vi "Init.vi"(8 "error in (no error)":errorcluster, 10 "Size":cluster{"Width":u16, "Height":u16}, 11 "Class 1 in":refnum<class "Freetype Drawer.lvclass">) -> (0 "error out":errorcluster, 3 "Class 1 out":refnum<class "Freetype Drawer.lvclass">)   [LabVIEW 2023, in "Freetype Drawer.lvlib" / "Freetype Drawer.lvclass"]
uses:
  Freetype Drawer.lvclass
  Freetype Drawer.lvclass/Freetype Drawer.ctl
  Freetype Drawer.lvlib
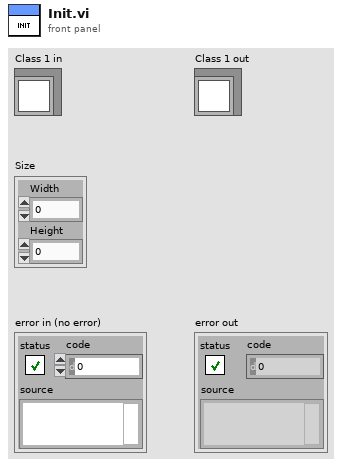
[diagram p1: front panel]
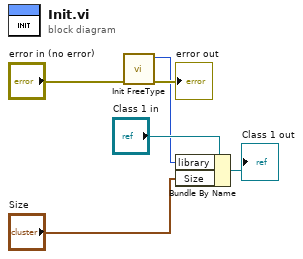
[diagram p0: block diagram]
diagram:
  n1 = call "Init FreeType.vi"("error in (no error)"="error in (no error)") -> ("error out"=→"error out":errorcluster, "library"=w2:i64)  [unwired: 9 in]
  n2 = Bundle By Name(cluster="Class 1 in", "library"=w2, "Size"="Size") -> (→"Class 1 out":refnum<class "Freetype Drawer.lvclass">)
